vi "rsscope_core_global.vi"() -> ()   [LabVIEW 2014] (continued)
waveform types you can assign a suitable color table:\n              - each waveform of any channel\n              - a reference waveform\n              - the results of a mathematical function\n              - a stored measurement\n              - an xy-diagram\n              The following default color tables are provided:\n              - &apos;Temperature&apos;: shade of color changes gradually from blue (low temperature) to red (high temperature) with increasing cumulative occurance.\n              - &apos;False colors&apos;: color changes gradually in a wide color spectrum with increasing cumulative occurance.\n              - Spectrum: colors used to display the wave lengths of the light are assigned to the cumulative occurance. High cumulative occurance is displayed blue like high wave lenght.\n              - Single event: single events and very seldom events appear yellow, a higher cumulative occurance is shown with blue color. This view helps to indentify specific events.\n\nAvailable Repeated Capabilities:\nWfmSuffix: WfmNone, WfmC1W1, WfmC1W2, WfmC1W3, WfmC2W1, WfmC2W2, WfmC2W3, WfmC3W1, WfmC3W2, WfmC3W3, WfmC4W1, WfmC4W2, WfmC4W3, WfmMath1, WfmMath2, WfmMath3, WfmMath4, WfmRef1, WfmRef2, WfmRef3, WfmRef4, WfmXY1, WfmXY2, WfmXY3, WfmXY4, WfmMeas1, WfmMeas2, WfmMeas3, WfmMeas4, WfmMeas5, WfmMeas6, WfmMeas7, WfmMeas8, WfmSbus1, WfmSbus2, WfmSbus3, WfmSbus4, WfmD0, WfmD1, WfmD2, WfmD3, WfmD4, WfmD5, WfmD6, WfmD7, WfmD8, WfmD9, WfmD10, WfmD11, WfmD12, WfmD13, WfmD14, WfmD15, WfmMSO1, WfmMSO2, WfmMSO3, WfmMSO4, WfmTRK1, WfmTRK2, WfmTRK3, WfmTRK4, WfmTRK5, WfmTRK6, WfmTRK7, WfmTRK8, WfmSpectrum1, WfmSpectrum2, WfmSpectrum3, WfmSpectrum4, WfmSG1TL1, WfmSG1TL2, WfmSG2TL1, WfmSG2TL2, WfmSG3TL1, WfmSG3TL2, WfmSG4TL1, WfmSG4TL2, WfmEye1, WfmEye2, WfmEye3, WfmEye4, WfmZ1V1, WfmZ1V2, WfmZ1V3, WfmZ1V4, WfmZ1I1, WfmZ1I2, WfmZ1I3, WfmZ1I4, WfmZ2V1, WfmZ2V2, WfmZ2V3, WfmZ2V4, WfmZ2I1, WfmZ2I2, WfmZ2I3, WfmZ2I4, WfmDiff1, WfmDiff2, WfmCommon1, WfmCommon2, WfmTDRZ, WfmTDRH, WfmTDRR, WfmMath5, WfmMath6, WfmMath7, WfmMath8, WfmSpectrum5, WfmSpectrum6, WfmSpectrum7, WfmSpectrum8, WfmSG5TL1, WfmSG5TL2, WfmSG6TL1, WfmSG6TL2, WfmSG7TL1, WfmSG7TL2, WfmSG8TL1, WfmSG8TL2, WfmHP1, WfmHP2, WfmHP3, WfmHP4, WfmHP5, WfmHP6, WfmHP7, WfmHP8, WfmHP9, WfmHP10, WfmBathtub1, WfmBathMeas1, WfmStepResp1, WfmSRHist1, WfmSDHist1, WfmTJHist1, WfmDJHist1, WfmDDJHist1, WfmPJHist1, WfmRJOHist1, WfmSRTrack1, WfmTJTrack1, WfmDJTrack1, WfmDDJTrack1, WfmPJTrack1, WfmRJTrack1, WfmTJSpectrum1, WfmDDJSpectrum1, WfmPJSpectrum1, WfmRJSpectrum1, WfmSEye1, WfmBathtub2, WfmBathMeas2, WfmStepResp2, WfmSRHist2, WfmSDHist2, WfmTJHist2, WfmDJHist2, WfmDDJHist2, WfmPJHist2, WfmRJOHist2, WfmSRTrack2, WfmSDTrack2, WfmTJTrack2, WfmDDJTrack2, WfmPJTrack2, WfmRJTrack2, WfmTJSpectrum2, WfmDDJSpectrum2, WfmPJSpectrum2, WfmRJSpectrum2, WfmSEye2, WfmNBathtub1, WfmNBathMeas1, WfmTNHist1, WfmDNHist1, WfmDDNHist1, WfmPNHist1, WfmRNOTrack1, WfmTNTrack1, WfmDDNTrack1, WfmPNTrack1, WfmRNTrack1, WfmTNSpectrum1, WfmDDNSpectrum1, WfmPNSpectrum1, WfmRNSpectrum1, WfmNBathtub2, WfmNBathMeas2, WfmTNHist2, WfmDNHist2, WfmDDNHist2, WfmPNHist2, WfmRNOHist2, WfmTNTrack2, WfmDDNTrack2, WfmPNTrack2, WfmRNTrack2, WfmTNSpectrum2, WfmDDNSpectrum2, WfmPNSpectrum2, WfmRNSpectrum2, WfmPJDHist1, WfmBUJHist1, WfmRJHist1, WfmPJDTrack1, WfmPJDSpectrum1, WfmPJDHist2, WfmBUJHist2, WfmRJHist2, WfmPJDTrack2, WfmPJDSpectrum2, WfmPNDHist1, WfmBUNHist1, WfmRNHist1, WfmPNDTrack1, WfmPNDSpectrum1, WfmPNDHist2, WfmBUNHist2, WfmRNHist2, WfmPNDTrack2, WfmPNDSpectrum2\r\n\nRemote-control command(s):\nDISPlay:COLor:SIGNal<m>:ASSign"}, {"Level"=4, "Class Only"=FALSE, "Identifier"="RSSCOPE_ATTR_SIGNAL_COLOR", "Descriptive Name"="Signal Color", "Data Type"=5, "Command"="DISP:COL:SIGN{WfmSuffix}:COL", "Access"=2, "Range Table"="RsScope_rngSignalColor", "Read Callback"="", "Write Callback"="", "Supported Models"="", "Instrument Options"="", "Flags"=0, "Help"="Decimal value of the ARGB color. Use the color dialog box on the instrument to get the hex value of the color, and convert the hex value to a decimal value.\n0 is fully transparent black.\n4278190080 (dec) = FF000000 (hex) is opaque black.\n4294967295 (dec) = FFFFFFFF (hex) is opaque white.\n\nAvailable Repeated Capabilities:\nWfmSuffix: WfmNone, WfmC1W1, WfmC1W2, WfmC1W3, WfmC2W1, WfmC2W2, WfmC2W3, WfmC3W1, WfmC3W2, WfmC3W3, WfmC4W1, WfmC4W2, WfmC4W3, WfmMath1, WfmMath2, WfmMath3, WfmMath4, WfmRef1, WfmRef2, WfmRef3, WfmRef4, WfmXY1, WfmXY2, WfmXY3, WfmXY4, WfmMeas1, WfmMeas2, WfmMeas3, WfmMeas4, WfmMeas5, WfmMeas6, WfmMeas7, WfmMeas8, WfmSbus1, WfmSbus2, WfmSbus3, WfmSbus4, WfmD0, WfmD1, WfmD2, WfmD3, WfmD4, WfmD5, WfmD6, WfmD7, WfmD8, WfmD9, WfmD10, WfmD11, WfmD12, WfmD13, WfmD14, WfmD15, WfmMSO1, WfmMSO2, WfmMSO3, WfmMSO4, WfmTRK1, WfmTRK2, WfmTRK3, WfmTRK4, WfmTRK5, WfmTRK6, WfmTRK7, WfmTRK8, WfmSpectrum1, WfmSpectrum2, WfmSpectrum3, WfmSpectrum4, WfmSG1TL1, WfmSG1TL2, WfmSG2TL1, WfmSG2TL2, WfmSG3TL1, WfmSG3TL2, WfmSG4TL1, WfmSG4TL2, WfmEye1, WfmEye2, WfmEye3, WfmEye4, WfmZ1V1, WfmZ1V2, WfmZ1V3, WfmZ1V4, WfmZ1I1, WfmZ1I2, WfmZ1I3, WfmZ1I4, WfmZ2V1, WfmZ2V2, WfmZ2V3, WfmZ2V4, WfmZ2I1, WfmZ2I2, WfmZ2I3, WfmZ2I4, WfmDiff1, WfmDiff2, WfmCommon1, WfmCommon2, WfmTDRZ, WfmTDRH, WfmTDRR, WfmMath5, WfmMath6, WfmMath7, WfmMath8, WfmSpectrum5, WfmSpectrum6, WfmSpectrum7, WfmSpectrum8, WfmSG5TL1, WfmSG5TL2, WfmSG6TL1, WfmSG6TL2, WfmSG7TL1, WfmSG7TL2, WfmSG8TL1, WfmSG8TL2, WfmHP1, WfmHP2, WfmHP3, WfmHP4, WfmHP5, WfmHP6, WfmHP7, WfmHP8, WfmHP9, WfmHP10, WfmBathtub1, WfmBathMeas1, WfmStepResp1, WfmSRHist1, WfmSDHist1, WfmTJHist1, WfmDJHist1, WfmDDJHist1, WfmPJHist1, WfmRJOHist1, WfmSRTrack1, WfmTJTrack1, WfmDJTrack1, WfmDDJTrack1, WfmPJTrack1, WfmRJTrack1, WfmTJSpectrum1, WfmDDJSpectrum1, WfmPJSpectrum1, WfmRJSpectrum1, WfmSEye1, WfmBathtub2, WfmBathMeas2, WfmStepResp2, WfmSRHist2, WfmSDHist2, WfmTJHist2, WfmDJHist2, WfmDDJHist2, WfmPJHist2, WfmRJOHist2, WfmSRTrack2, WfmSDTrack2, WfmTJTrack2, WfmDDJTrack2, WfmPJTrack2, WfmRJTrack2, WfmTJSpectrum2, WfmDDJSpectrum2, WfmPJSpectrum2, WfmRJSpectrum2, WfmSEye2, WfmNBathtub1, WfmNBathMeas1, WfmTNHist1, WfmDNHist1, WfmDDNHist1, WfmPNHist1, WfmRNOTrack1, WfmTNTrack1, WfmDDNTrack1, WfmPNTrack1, WfmRNTrack1, WfmTNSpectrum1, WfmDDNSpectrum1, WfmPNSpectrum1, WfmRNSpectrum1, WfmNBathtub2, WfmNBathMeas2, WfmTNHist2, WfmDNHist2, WfmDDNHist2, WfmPNHist2, WfmRNOHist2, WfmTNTrack2, WfmDDNTrack2, WfmPNTrack2, WfmRNTrack2, WfmTNSpectrum2, WfmDDNSpectrum2, WfmPNSpectrum2, WfmRNSpectrum2, WfmPJDHist1, WfmBUJHist1, WfmRJHist1, WfmPJDTrack1, WfmPJDSpectrum1, WfmPJDHist2, WfmBUJHist2, WfmRJHist2, WfmPJDTrack2, WfmPJDSpectrum2, WfmPNDHist1, WfmBUNHist1, WfmRNHist1, WfmPNDTrack1, WfmPNDSpectrum1, WfmPNDHist2, WfmBUNHist2, WfmRNHist2, WfmPNDTrack2, WfmPNDSpectrum2\r\n\nRemote-control command(s):\nDISPlay:COLor:SIGNal<m>:COLor"}, {"Level"=2, "Class Only"=TRUE, "Identifier"="", "Descriptive Name"="Color Tables", "Data Type"=0, "Command"="", "Access"=0, "Range Table"="", "Read Callback"="", "Write Callback"="", "Supported Models"="", "Instrument Options"="", "Flags"=0, "Help"="Configuration for color tables."}, {"Level"=3, "Class Only"=FALSE, "Identifier"="RSSCOPE_ATTR_ADD_COLOR_TABLE", "Descriptive Name"="Add Color Table", "Data Type"=2, "Command"="DISP:COL:PAL:ADD", "Access"=1, "Range Table"="", "Read Callback"="", "Write Callback"="", "Supported Models"="", "Instrument Options"="", "Flags"=0, "Help"="Adds a new color table with the specified name.\n\nAvailable Repeated Capabilities:\nNone\n\nRemote-control command(s):\nDISPlay:COLor:PALette:ADD"}, {"Level"=3, "Class Only"=FALSE, "Identifier"="RSSCOPE_ATTR_REMOVE_COLOR_TABLE", "Descriptive Name"="Remove Color Table", "Data Type"=2, "Command"="DISP:COL:PAL:REM", "Access"=1, "Range Table"="", "Read Callback"="", "Write Callback"="", "Supported Models"="", "Instrument Options"="", "Flags"=0, "Help"="Removes the specified color table.\n\nAvailable Repeated Capabilities:\nNone\n\nRemote-control command(s):\nDISPlay:COLor:PALette:REMove"}, {"Level"=3, "Class Only"=FALSE, "Identifier"="RSSCOPE_ATTR_COLOR_TABLE_COUNT", "Descriptive Name"="Color Table Count", "Data Type"=0, "Command"="DISP:COL:PAL:COUN?", "Access"=0, "Range Table"="", "Read Callback"="", "Write Callback"="", "Supported Models"="", "Instrument Options"="", "Flags"=0, "Help"="Queries the number of configured color maps.\n\nAvailable Repeated Capabilities:\nNone\n\nRemote-control command(s):\nDISPlay:COLor:PALette:COUNt?"}, {"Level"=3, "Class Only"=FALSE, "Identifier"="RSSCOPE_ATTR_COLOR_TABLE_APPEND_NEW_ROW", "Descriptive Name"="Color Table Append New Row", "Data Type"=2, "Command"="DISP:COL:PAL:POIN:ADD", "Access"=1, "Range Table"="", "Read Callback"="", "Write Callback"="", "Supported Models"="", "Instrument Options"="", "Flags"=0, "Help"="Appends a new row at the end of the color table.\n\nAvailable Repeated Capabilities:\nNone\n\nRemote-control command(s):\nDISPlay:COLor:PALette:POINt:ADD"}, {"Level"=2, "Class Only"=TRUE, "Identifier"="", "Descriptive Name"="Diagram Layout", "Data Type"=0, "Command"="", "Access"=0, "Range Table"="", "Read Callback"="", "Write Callback"="", "Supported Models"="", "Instrument Options"="", "Flags"=0, "Help"="Configuration for diagram layout."}, {"Level"=3, "Class Only"=FALSE, "Identifier"="RSSCOPE_ATTR_DIAGRAM_SHOW_GRID", "Descriptive Name"="Diagram Show Grid", "Data Type"=3, "Command"="DISP:DIAG:GRID", "Access"=2, "Range Table"="", "Read Callback"="", "Write Callback"="", "Supported Models"="", "Instrument Options"="", "Flags"=0, "Help"="If enabled, a grid is displayed in the diagram area.\n\nAvailable Repeated Capabilities:\nNone\n\nRemote-control command(s):\nDISPlay:DIAGram:GRID"}, {"Level"=3, "Class Only"=FALSE, "Identifier"="RSSCOPE_ATTR_DIAGRAM_SHOW_CROSSHAIR", "Descriptive Name"="Diagram Show Crosshair", "Data Type"=3, "Command"="DISP:DIAG:CROS", "Access"=2, "Range Table"="", "Read Callback"="", "Write Callback"="", "Supported Models"="", "Instrument Options"="", "Flags"=0, "Help"="If selected, a crosshair is displayed in the diagram area. A crosshair allows you to select a specific data point by its co-ordinates.\n\nAvailable Repeated Capabilities:\nNone\n\nRemote-control command(s):\nDISPlay:DIAGram:CROSshair"}, {"Level"=3, "Class Only"=FALSE, "Identifier"="RSSCOPE_ATTR_DIAGRAM_SHOW_LABELS", "Descriptive Name"="Diagram Show Labels", "Data Type"=3, "Command"="DISP:DIAG:LAB", "Access"=2, "Range Table"="", "Read Callback"="", "Write Callback"="", "Supported Models"="", "Instrument Options"="", "Flags"=0, "Help"="If enabled, labels mark values on the x- and y-axes in specified intervals in the diagram.\n\nAvailable Repeated Capabilities:\nNone\n\nRemote-control command(s):\nDISPlay:DIAGram:LABels"}, {"Level"=3, "Class Only"=FALSE, "Identifier"="RSSCOPE_ATTR_DIAGRAM_SHOW_TAB_TITLES", "Descriptive Name"="Diagram Show Tab Titles", "Data Type"=3, "Command"="DISP:DIAG:TITL", "Access"=2, "Range Table"="", "Read Callback"="", "Write Callback"="", "Supported Models"="", "Instrument Options"="", "Flags"=0, "Help"="If enabled, the tab titles of all diagrams are displayed: &apos;Diagram1&apos;, &apos;Diagram2&apos;, ...\nIf disabled, the tab titles are not shown except for those in a tabbed diagram. In tabbed diagrams, the tab titles are required to change the tabs.\n\nAvailable Repeated Capabilities:\nNone\n\nRemote-control command(s):\nDISPlay:DIAGram:TITLe"}, {"Level"=3, "Class Only"=FALSE, "Identifier"="RSSCOPE_ATTR_DIAGRAM_KEEP_Y_GRID_FIXED", "Descriptive Name"="Diagram Keep Y-grid Fixed", "Data Type"=3, "Command"="DISP:DIAG:YFIX", "Access"=2, "Range Table"="", "Read Callback"="", "Write Callback"="", "Supported Models"="", "Instrument Options"="", "Flags"=0, "Help"="If enabled, the horizontal grid lines remain in their position when the position of the curve is changed. Only the values at the grid lines are adapted. This reflects the behavior of traditional oscilloscopes.\n\nAvailable Repeated Capabilities:\nNone\n\nRemote-control command(s):\nDISPlay:DIAGram:YFIXed"}, {"Level"=3, "Class Only"=FALSE, "Identifier"="RSSCOPE_ATTR_DIAGRAM_KEEP_X_GRID_FIXED", "Descriptive Name"="Diagram Keep X-grid Fixed", "Data Type"=3, "Command"="DISP:DIAG:XFIX", "Access"=2, "Range Table"="", "Read Callback"="", "Write Callback"="", "Supported Models"="", "Instrument Options"="", "Flags"=0, "Help"="If enabled, the vertical grid lines remain in their position when the horizontal position is changed. Only the values at the grid lines are adapted.\n\nAvailable Repeated Capabilities:\nNone\n\nRemote-control command(s):\nDISPlay:DIAGram:XFIXed"}, {"Level"=3, "Class Only"=FALSE, "Identifier"="RSSCOPE_ATTR_DIAGRAM_SHOW_FINE_GRID_SCALE", "Descriptive Name"="Diagram Show Fine Grid Scale", "Data Type"=3, "Command"="DISP:DIAG:FIN", "Access"=2, "Range Table"="", "Read Callback"="", "Write Callback"="", "Supported Models"="", "Instrument Options"="", "Flags"=0, "Help"="Configures fine grid scaling.\n\nAvailable Repeated Capabilities:\nNone\n\nRemote-control command(s):\nDISPlay:DIAGram:FINegrid"}, {"Level"=3, "Class Only"=FALSE, "Identifier"="RSSCOPE_ATTR_SIGNAL_BAR_STATE", "Descriptive Name"="Signal Bar State", "Data Type"=3, "Command"="DISP:SIGB:STAT", "Access"=2, "Range Table"="", "Read Callback"="", "Write Callback"="", "Supported Models"="", "Instrument Options"="", "Flags"=0, "Help"="If enabled, the signal bar is displayed in the diagram area.\n\nAvailable Repeated Capabilities:\nNone\n\nRemote-control command(s):\nDISPlay:SIGBar[:STATe]"}, {"Level"=3, "Class Only"=FALSE, "Identifier"="RSSCOPE_ATTR_SIGNAL_BAR_POSITION", "Descriptive Name"="Signal Bar Position", "Data Type"=0, "Command"="DISP:SIGB:POS", "Access"=2, "Range Table"="rsscope_rngSignalBarPostion", "Read Callback"="", "Write Callback"="", "Supported Models"="", "Instrument Options"="", "Flags"=0, "Help"="The signal bar can be placed vertically at the right (default position) or at the left, or horizontally at the top, bottom or center of the diagram to ensure best visibility of the waveforms.\n\nAvailable Repeated Capabilities:\nNone\n\nRemote-control command(s):\nDISPlay:SIGBar:POSition"}, {"Level"=3, "Class Only"=FALSE, "Identifier"="RSSCOPE_ATTR_SIGNAL_BAR_AUTO_HIDE", "Descriptive Name"="Signal Bar Auto Hide", "Data Type"=3, "Command"="DISP:SIGB:HIDE:AUTO", "Access"=2, "Range Table"="", "Read Callback"="", "Write Callback"="", "Supported Models"="", "Instrument Options"="", "Flags"=0, "Help"="If enabled, the signal bar disappears automatically after some time, similar to the Windows task bar. With the commands DISPlay:SIGBar:HIDE:TIME and DISPlay:SIGBar:HIDE:OPACity, you can define when and how the signal bar hides.\nThe signal bar reappears if you tap it, or if an action changes the content of the bar.\n\nAvailable Repeated Capabilities:\nNone\n\nRemote-control command(s):\nDISPlay:SIGBar:HIDE[:AUTO]"}, {"Level"=3, "Class Only"=FALSE, "Identifier"="RSSCOPE_ATTR_SIGNAL_BAR_HIDE_TIME", "Descriptive Name"="Signal Bar Hide Time", "Data Type"=1, "Command"="DISP:SIGB:HIDE:TIME", "Access"=2, "Range Table"="rsscope_rngSignalBarHideTime", "Read Callback"="", "Write Callback"="", "Supported Models"="", "Instrument Options"="", "Flags"=0, "Help"="Sets the time when the signal bar is faded out if DISPlay:SIGBar:HIDE[:AUTO] is &apos;ON&apos;\n\nAvailable Repeated Capabilities:\nNone\n\nRemote-control command(s):\nDISPlay:SIGBar:HIDE:TIME"}, {"Level"=3, "Class Only"=FALSE, "Identifier"="RSSCOPE_ATTR_SIGNAL_BAR_HIDE_HEAD", "Descriptive Name"="Signal Bar Hide Head", "Data Type"=3, "Command"="DISP:SIGB:HIDE:HEAD", "Access"=2, "Range Table"="", "Read Callback"="", "Write Callback"="", "Supported Models"="", "Instrument Options"="", "Flags"=0, "Help"="If enabled, the &apos;Auto hide&apos; function hides also the horizontal and trigger label at the top of the signal bar.\n\nAvailable Repeated Capabilities:\nNone\n\nRemote-control command(s):\nDISPlay:SIGBar:HIDE:HEAD"}, {"Level"=3, "Class Only"=FALSE, "Identifier"="RSSCOPE_ATTR_SIGNAL_BAR_HIDING_TRANSPARENCY", "Descriptive Name"="Signal Bar Hiding Transparency", "Data Type"=1, "Command"="DISP:SIGB:HIDE:TRAN", "Access"=2, "Range Table"="rsscope_rngSignalBarHidingTransparency", "Read Callback"="", "Write Callback"="", "Supported Models"="", "Instrument Options"="", "Flags"=0, "Help"="Sets the opacity, or transparency, of the signal bar. The minimum value is 30% for the least visibility of the signal bar, the maximum value is 80%.\n\nAvailable Repeated Capabilities:\nNone\n\nRemote-control command(s):\nDISPlay:SIGBar:HIDE:TRANsparency"}, {"Level"=3, "Class Only"=FALSE, "Identifier"="RSSCOPE_ATTR_SIGNAL_BAR_BORDER_COLOR", "Descriptive Name"="Signal Bar Border Color", "Data Type"=0, "Command"="DISP:SIGB:COL:BORD", "Access"=2, "Range Table"="", "Read Callback"="", "Write Callback"="", "Supported Models"="", "Instrument Options"="", "Flags"=0, "Help"="Defines the color of the signal bar border.\n\nAvailable Repeated Capabilities:\nNone\n\nRemote-control command(s):\nDISPlay:SIGBar:COLor:BORDer"}, {"Level"=3, "Class Only"=FALSE, "Identifier"="RSSCOPE_ATTR_SIGNAL_BAR_FILL_COLOR", "Descriptive Name"="Signal Bar Fill Color", "Data Type"=0, "Command"="DISP:SIGB:COL:FILL", "Access"=2, "Range Table"="", "Read Callback"="", "Write Callback"="", "Supported Models"="", "Instrument Options"="", "Flags"=0, "Help"="Define the fill color of the signal bar.\n\nAvailable Repeated Capabilities:\nNone\n\nRemote-control command(s):\nDISPlay:SIGBar:COLor:FILL"}, {"Level"=3, "Class Only"=FALSE, "Identifier"="RSSCOPE_ATTR_RESULT_BOX_POSITION", "Descriptive Name"="Result Box Position", "Data Type"=0, "Command"="DISP:RES:DEF", "Access"=2, "Range Table"="rsscope_rngResultBoxPosition", "Read Callback"="", "Write Callback"="", "Supported Models"="", "Instrument Options"="", "Flags"=0, "Help"="Defines where a new result box opens.\n\nAvailable Repeated Capabilities:\nNone\n\nRemote-control command(s):\nDISPlay:RESultboxes:DEFaultpos"}, {"Level"=3, "Class Only"=FALSE, "Identifier"="RSSCOPE_ATTR_REMOVE_DIAGRAM", "Descriptive Name"="Remove Diagram", "Data Type"=2, "Command"="LAY:REM", "Access"=1, "Range Table"="", "Read Callback"="", "Write Callback"="", "Supported Models"="", "Instrument Options"="", "Flags"=0, "Help"="Removes diagram\n\nAvailable Repeated Capabilities:\nNone\n\nRemote-control command(s):\nLAYout:REMove"}, {"Level"=3, "Class Only"=FALSE, "Identifier"="RSSCOPE_ATTR_DISPLAY_DIAGRAM", "Descriptive Name"="Display Diagram", "Data Type"=2, "Command"="LAY:SHOW", "Access"=1, "Range Table"="", "Read Callback"="", "Write Callback"="", "Supported Models"="", "Instrument Options"="", "Flags"=0, "Help"="Displays diagram.\n\nAvailable Repeated Capabilities:\nNone\n\nRemote-control command(s):\nLAYout:SHOW"}, {"Level"=3, "Class Only"=FALSE, "Identifier"="RSSCOPE_ATTR_REMOVE_WAVEFORM_FROM_DIAGRAM", "Descriptive Name"="Remove Waveform From Diagram", "Data Type"=0, "Command"="LAY:SIGN:UNAS", "Access"=1, "Range Table"="rsscope_rngWaveformParameter", "Read Callback"="", "Write Callback"="", "Supported Models"="", "Instrument Options"="", "Flags"=0, "Help"="Removes the specified waveform from the diagram.\n\nAvailable Repeated Capabilities:\nNone\n\nRemote-control command(s):\nLAYout:SIGNal:UNASsign"}, {"Level"=2, "Class Only"=TRUE, "Identifier"="", "Descriptive Name"="Waveform Label", "Data Type"=0, "Command"="", "Access"=0, "Range Table"="", "Read Callback"="", "Write Callback"="", "Supported Models"="", "Instrument Options"="", "Flags"=0, "Help"="Attributes which configures labels of waveforms."}, {"Level"=3, "Class Only"=FALSE, "Identifier"="RSSCOPE_ATTR_SELECTED_LABEL_NAME", "Descriptive Name"="Selected Label Name", "Data Type"=2, "Command"="", "Access"=2, "Range Table"="", "Read Callback"="", "Write Callback"="", "Supported Models"="", "Instrument Options"="", "Flags"=0, "Help"="This attribute selects the label name used for following attributes.\n\nAvailable Repeated Capabilities:\nNone\n\nRemote-control command(s):\ncmd"}, {"Level"=3, "Class Only"=FALSE, "Identifier"="RSSCOPE_ATTR_SELECTED_LABEL_SOURCE", "Descriptive Name"="Selected Label Source", "Data Type"=0, "Command"="", "Access"=2, "Range Table"="rsscope_rngWaveformParameter", "Read Callback"="", "Write Callback"="", "Supported Models"="", "Instrument Options"="", "Flags"=0, "Help"="Sets selector repeated capability Source.\n\nAvailable Repeated Capabilities:\nNone\n\nRemote-control command(s):\n"}, {"Level"=3, "Class Only"=FALSE, "Identifier"="RSSCOPE_ATTR_LABEL_SHOW", "Descriptive Name"="Label Show", "Data Type"=3, "Command"="DISP:SIGN:LAB:SHOW", "Access"=2, "Range Table"="", "Read Callback"="rsscope_FormatLabelSourceBoolean_ReadCallback.vi", "Write Callback"="rsscope_FormatLabelSourceBoolean_WriteCallback.vi", "Supported Models"="", "Instrument Options"="", "Flags"=0, "Help"="Selects the source for the label display and enables it.\n\nAvailable Repeated Capabilities:\nNone\n\nRemote-control command(s):\nDISPlay:SIGNal:LABel:SHOW"}, {"Level"=3, "Class Only"=FALSE, "Identifier"="RSSCOPE_ATTR_WAVEFORM_LABEL_FONT_SIZE", "Descriptive Name"="Waveform Label Font Size", "Data Type"=0, "Command"="DISPlay:SIGNal:LABel:FONTsize", "Access"=2, "Range Table"="RsScope_rngWaveformLabelFontSize", "Read Callback"="", "Write Callback"="", "Supported Models"="", "Instrument Options"="", "Flags"=0, "Help"="Sets the font size of waveform labels.\n\nAvailable Repeated Capabilities:\nNone\n\nRemote-control command(s):\nDISPlay:SIGNal:LABel:FONTsize"}, {"Level"=2, "Class Only"=TRUE, "Identifier"="", "Descriptive Name"="Zoom", "Data Type"=0, "Command"="", "Access"=0, "Range Table"="", "Read Callback"="", "Write Callback"="", "Supported Models"="", "Instrument Options"="", "Flags"=0, "Help"="The zoom attributes allow you to magnify a specific section of the diagram in order to view more details. You can define several zoom areas for the same diagram and even couple them, or you use the hardware zoom."}, {"Level"=3, "Class Only"=FALSE, "Identifier"="RSSCOPE_ATTR_DIAGRAM_ZOOM_OVERLAY", "Descriptive Name"="Diagram Zoom Overlay", "Data Type"=3, "Command"="LAY:ZOOM:ONED", "Access"=2, "Range Table"="", "Read Callback"="", "Write Callback"="", "Supported Models"="", "Instrument Options"="", "Flags"=0, "Help"="Shows all zooms of a diagram in one zoom window.\n\nAvailable Repeated Capabilities:\nNone\n\nRemote-control command(s):\nLAYout:ZOOM:ONEDiagram"}, {"Level"=2, "Class Only"=TRUE, "Identifier"="", "Descriptive Name"="XY Diagram", "Data Type"=0, "Command"="", "Access"=0, "Range Table"="", "Read Callback"="", "Write Callback"="", "Supported Models"="", "Instrument Options"="", "Flags"=0, "Help"="Configuration for XY diagrams."}, {"Level"=3, "Class Only"=FALSE, "Identifier"="RSSCOPE_ATTR_XY_DIAGRAM_STATE", "Descriptive Name"="XY Diagram State", "Data Type"=3, "Command"="WAV{XYDiagram}:XYC:STAT", "Access"=2, "Range Table"="", "Read Callback"="", "Write Callback"="", "Supported Models"="", "Instrument Options"="", "Flags"=0, "Help"="Activates an XY-waveform.\n\nAvailable Repeated Capabilities:\nXYDiagram: XY1, XY2, XY3, XY4\r\n\nRemote-control command(s):\nWAVeform<m>:XYCurve:STATe"}, {"Level"=3, "Class Only"=FALSE, "Identifier"="RSSCOPE_ATTR_XY_DIAGRAM_RATIO", "Descriptive Name"="XY Diagram Ratio", "Data Type"=3, "Command"="WAV{XYDiagram}:XYC:RAT", "Access"=2, "Range Table"="", "Read Callback"="", "Write Callback"="", "Supported Models"="", "Instrument Options"="", "Flags"=0, "Help"="If enabled, the x- and y-axes maintain a constant ratio in the diagram.\n\nAvailable Repeated Capabilities:\nXYDiagram: XY1, XY2, XY3, XY4\r\n\nRemote-control command(s):\nWAVeform<m>:XYCurve:RATio"}, {"Level"=3, "Class Only"=FALSE, "Identifier"="RSSCOPE_ATTR_SWAP_XY_DIAGRAM", "Descriptive Name"="Swap XY Diagram", "Data Type"=4, "Command"="WAV{XYDiagram}:XYC:SWAP", "Access"=1, "Range Table"="", "Read Callback"="", "Write Callback"="", "Supported Models"="", "Instrument Options"="", "Flags"=0, "Help"="Replaces the source of the x-axis with the source of the y-axis and vice versa.\n\nAvailable Repeated Capabilities:\nXYDiagram: XY1, XY2, XY3, XY4\r\n\nRemote-control command(s):\nWAVeform<m>:XYCurve:SWAP"}, {"Level"=3, "Class Only"=FALSE, "Identifier"="RSSCOPE_ATTR_XY_DIAGRAM_X_SOURCE", "Descriptive Name"="XY Diagram X Source", "Data Type"=0, "Command"="WAV{XYDiagram}:XYC:XSO", "Access"=2, "Range Table"="rsscope_rngWaveformParameterXY", "Read Callback"="", "Write Callback"="", "Supported Models"="", "Instrument Options"="", "Flags"=0, "Help"="Defines the signal source that supplies the x-values of the XY-diagram.\n\nAvailable Repeated Capabilities:\nXYDiagram: XY1, XY2, XY3, XY4\r\n\nRemote-control command(s):\nWAVeform<m>:XYCurve:XSOurce"}, {"Level"=3, "Class Only"=FALSE, "Identifier"="RSSCOPE_ATTR_XY_DIAGRAM_Y_SOURCE", "Descriptive Name"="XY Diagram Y Source", "Data Type"=0, "Command"="WAV{XYDiagram}:XYC:YSO", "Access"=2, "Range Table"="rsscope_rngWaveformParameterXY", "Read Callback"="", "Write Callback"="", "Supported Models"="", "Instrument Options"="", "Flags"=0, "Help"="Defines the signal source that supplies the y-values of the XY-diagram.\n\nAvailable Repeated Capabilities:\nXYDiagram: XY1, XY2, XY3, XY4\r\n\nRemote-control command(s):\nWAVeform<m>:XYCurve:YSOurce"}, {"Level"=2, "Class Only"=TRUE, "Identifier"="", "Descriptive Name"="History", "Data Type"=0, "Command"="", "Access"=0, "Range Table"="", "Read Callback"="", "Write Callback"="", "Supported Models"="", "Instrument Options"="", "Flags"=0, "Help"="This class contains functions for history viewing and information."}, {"Level"=3, "Class Only"=FALSE, "Identifier"="RSSCOPE_ATTR_HISTORY_GET_ACQUISITIONS_COUNT", "Descriptive Name"="History Get Acquisitions Count", "Data Type"=0, "Command"="ACQ:AVA?", "Access"=0, "Range Table"="", "Read Callback"="", "Write Callback"="", "Supported Models"="", "Instrument Options"="", "Flags"=0, "Help"="Returns the number of acquisitions currently saved in the memory.\n\nAvailable Repeated Capabilities:\nNone\n\nRemote-control command(s):\nACQuire:AVAilable?"}, {"Level"=3, "Class Only"=TRUE, "Identifier"="", "Descriptive Name"="Channel", "Data Type"=0, "Command"="", "Access"=0, "Range Table"="", "Read Callback"="", "Write Callback"="", "Supported Models"="", "Instrument Options"="", "Flags"=0, "Help"="Configures Display History properties."}, {"Level"=4, "Class Only"=TRUE, "Identifier"="", "Descriptive Name"="Waveform", "Data Type"=0, "Command"="", "Access"=0, "Range Table"="", "Read Callback"="", "Write Callback"="", "Supported Models"="", "Instrument Options"="", "Flags"=0, "Help"="Configures History Waveform properties."}, {"Level"=5, "Class Only"=FALSE, "Identifier"="RSSCOPE_ATTR_HISTORY_STATE", "Descriptive Name"="History State", "Data Type"=3, "Command"="CHAN{Channel}:WAV{Waveform}:HIST", "Access"=2, "Range Table"="", "Read Callback"="", "Write Callback"="", "Supported Models"="", "Instrument Options"="", "Flags"=0, "Help"="Enables or disables the history display.\n\nAvailable Repeated Capabilities:\nChannel: CH1, CH2, CH3, CH4, CHExt\r\nWaveform: W0, W1, W2, W3\r\n\nRemote-control command(s):\nCHANnel<m>[:WAVeform<n>]:HISTory[:STATe]"}, {"Level"=5, "Class Only"=FALSE, "Identifier"="RSSCOPE_ATTR_HISTORY_START_INDEX", "Descriptive Name"="History Start Index", "Data Type"=0, "Command"="CHAN{Channel}:WAV{Waveform}:HIST:STAR", "Access"=2, "Range Table"="", "Read Callback"="", "Write Callback"="", "Supported Models"="", "Instrument Options"="", "Flags"=0, "Help"="Sets the start point for the history replay.\nNote: The &apos;Start index&apos; is always negative.\n\nAvailable Repeated Capabilities:\nChannel: CH1, CH2, CH3, CH4, CHExt\r\nWaveform: W0, W1, W2, W3\r\n\nRemote-control command(s):\nCHANnel<m>[:WAVeform<n>]:HISTory:STARt"}, {"Level"=5, "Class Only"=FALSE, "Identifier"="RSSCOPE_ATTR_HISTORY_STOP_INDEX", "Descriptive Name"="History Stop Index", "Data Type"=0, "Command"="CHAN{Channel}:WAV{Waveform}:HIST:STOP", "Access"=2, "Range Table"="", "Read Callback"="", "Write Callback"="", "Supported Models"="", "Instrument Options"="", "Flags"=0, "Help"="Sets the end point for the history viewer.\nNote: The newest acquisition always has the index &apos;0&apos;.\n\nAvailable Repeated Capabilities:\nChannel: CH1, CH2, CH3, CH4, CHExt\r\nWaveform: W0, W1, W2, W3\r\n\nRemote-control command(s):\nCHANnel<m>[:WAVeform<n>]:HISTory:STOP"}, {"Level"=5, "Class Only"=FALSE, "Identifier"="RSSCOPE_ATTR_HISTORY_ACQUISITION_VIEW", "Descriptive Name"="History Acquisition View", "Data Type"=0, "Command"="CHAN{Channel}:WAV{Waveform}:HIST:CURR", "Access"=2, "Range Table"="", "Read Callback"="", "Write Callback"="", "Supported Models"="", "Instrument Options"="", "Flags"=0, "Help"="Selects a particular acquisition in the memory to display it.\n\nAvailable Repeated Capabilities:\nChannel: CH1, CH2, CH3, CH4, CHExt\r\nWaveform: W0, W1, W2, W3\r\n\nRemote-control command(s):\nCHANnel<m>[:WAVeform<n>]:HISTory:CURRent"}, {"Level"=5, "Class Only"=FALSE, "Identifier"="RSSCOPE_ATTR_HISTORY_ACQUISITION_TIME", "Descriptive Name"="History Acquisition Time", "Data Type"=1, "Command"="CHAN{Channel}:WAV{Waveform}:HIST:TPAC", "Access"=2, "Range Table"="rsscope_rngHistAcqTime", "Read Callback"="", "Write Callback"="", "Supported Models"="", "Instrument Options"="", "Flags"=0, "Help"="Sets the display time for one acquisition.\n\nAvailable Repeated Capabilities:\nChannel: CH1, CH2, CH3, CH4, CHExt\r\nWaveform: W0, W1, W2, W3\r\n\nRemote-control command(s):\nCHANnel<m>[:WAVeform<n>]:HISTory:TPACq"}, {"Level"=5, "Class Only"=FALSE, "Identifier"="RSSCOPE_ATTR_HISTORY_AUTO_REPEAT", "Descriptive Name"="History Auto Repeat", "Data Type"=3, "Command"="CHAN{Channel}:WAV{Waveform}:HIST:REPL", "Access"=2, "Range Table"="", "Read Callback"="", "Write Callback"="", "Supported Models"="", "Instrument Options"="", "Flags"=0, "Help"="Sets if the replay of the history waveform sequence repeats automatically.\n\nAvailable Repeated Capabilities:\nChannel: CH1, CH2, CH3, CH4, CHExt\r\nWaveform: W0, W1, W2, W3\r\n\nRemote-control command(s):\nCHANnel<m>[:WAVeform<n>]:HISTory:REPLay"}, {"Level"=5, "Class Only"=FALSE, "Identifier"="RSSCOPE_ATTR_HISTORY_PLAYBACK", "Descriptive Name"="History Playback", "Data Type"=4, "Command"="CHAN{Channel}:WAV{Waveform}:HIST:PLAY", "Access"=1, "Range Table"="", "Read Callback"="", "Write Callback"="", "Supported Models"="", "Instrument Options"="", "Flags"=0, "Help"="Starts and stops the replay of the history waveforms.\n\nAvailable Repeated Capabilities:\nChannel: CH1, CH2, CH3, CH4, CHExt\r\nWaveform: W0, W1, W2, W3\r\n\nRemote-control command(s):\nCHANnel<m>[:WAVeform<n>]:HISTory:PLAY"}, {"Level"=5, "Class Only"=FALSE, "Identifier"="RSSCOPE_ATTR_HISTORY_ABSOLUTE_TIME_STAMP", "Descriptive Name"="History Absolute Time Stamp", "Data Type"=2, "Command"="CHAN{Channel}:WAV{Waveform}:HIST:TSAB?", "Access"=0, "Range Table"="", "Read Callback"="", "Write Callback"="", "Supported Models"="", "Instrument Options"="", "Flags"=0, "Help"="Returns the abolsute daytime of the current acquisition that is shown in the history viewer\n\nAvailable Repeated Capabilities:\nChannel: CH1, CH2, CH3, CH4, CHExt\r\nWaveform: W0, W1, W2, W3\r\n\nRemote-control command(s):\nCHANnel<m>[:WAVeform<n>]:HISTory:TSABsolute?"}, {"Level"=5, "Class Only"=FALSE, "Identifier"="RSSCOPE_ATTR_HISTORY_RELATIVE_TIME_STAMP", "Descriptive Name"="History Relative Time Stamp", "Data Type"=2, "Command"="CHAN{Channel}:WAV{Waveform}:HIST:TSR?", "Access"=0, "Range Table"="", "Read Callback"="", "Write Callback"="", "Supported Models"="", "Instrument Options"="", "Flags"=0, "Help"="Returns the relative time of the current acquisition - the time difference to the newest acquisition (index = 0).\n\nAvailable Repeated Capabilities:\nChannel: CH1, CH2, CH3, CH4, CHExt\r\nWaveform: W0, W1, W2, W3\r\n\nRemote-control command(s):\nCHANnel<m>[:WAVeform<n>]:HISTory:TSRelative?"}, {"Level"=5, "Class Only"=FALSE, "Identifier"="RSSCOPE_ATTR_HISTORY_TIME_REFERENCE", "Descriptive Name"="History Time Reference", "Data Type"=1, "Command"="CHAN{Channel}:WAV{Waveform}:HIST:TSRR?", "Access"=0, "Range Table"="", "Read Callback"="", "Write Callback"="", "Supported Models"="", "Instrument Options"="", "Flags"=0, "Help"="Returns the relative time of the currently selected acquisition and the internal reference time (horizontal alignment) in history view with respect to the acquisition with index 0.\n\nAvailable Repeated Capabilities:\nChannel: CH1, CH2, CH3, CH4, CHExt\r\nWaveform: W0, W1, W2, W3\r\n\nRemote-control command(s):\nCHANnel<m>[:WAVeform<n>]:HISTory:TSRReference?"}, {"Level"=5, "Class Only"=FALSE, "Identifier"="RSSCOPE_ATTR_HISTORY_DATE", "Descriptive Name"="History Date", "Data Type"=2, "Command"="CHAN{Channel}:WAV{Waveform}:HIST:TSD?", "Access"=0, "Range Table"="", "Read Callback"="", "Write Callback"="", "Supported Models"="", "Instrument Options"="", "Flags"=0, "Help"="Returns the date of the current acquisition that is shown in the history viewer.\n\nAvailable Repeated Capabilities:\nChannel: CH1, CH2, CH3, CH4, CHExt\r\nWaveform: W0, W1, W2, W3\r\n\nRemote-control command(s):\nCHANnel<m>[:WAVeform<n>]:HISTory:TSDate?"}, {"Level"=1, "Class Only"=TRUE, "Identifier"="", "Descriptive Name"="Data Management", "Data Type"=0, "Command"="", "Access"=0, "Range Table"="", "Read Callback"="", "Write Callback"="", "Supported Models"="", "Instrument Options"="", "Flags"=0, "Help"="Mass memory, save and load"}, {"Level"=2, "Class Only"=FALSE, "Identifier"="RSSCOPE_ATTR_SAVE", "Descriptive Name"="Save", "Data Type"=0, "Command"="*SAV", "Access"=1, "Range Table"="", "Read Callback"="", "Write Callback"="", "Supported Models"="", "Instrument Options"="", "Flags"=0, "Help"="Saves settings.\n\nAvailable Repeated Capabilities:\nNone\n\nRemote-control command(s):\n*SAV"}, {"Level"=2, "Class Only"=FALSE, "Identifier"="RSSCOPE_ATTR_RECALL", "Descriptive Name"="Recall", "Data Type"=0, "Command"="*RCL", "Access"=1, "Range Table"="", "Read Callback"="", "Write Callback"="", "Supported Models"="", "Instrument Options"="", "Flags"=0, "Help"="Recalls settings.\n\nAvailable Repeated Capabilities:\nNone\n\nRemote-control command(s):\n*RCL"}, {"Level"=2, "Class Only"=FALSE, "Identifier"="RSSCOPE_ATTR_DRIVES", "Descriptive Name"="Drives", "Data Type"=2, "Command"="MMEM:DRIV?", "Access"=0, "Range Table"="", "Read Callback"="", "Write Callback"="", "Supported Models"="", "Instrument Options"="", "Flags"=0, "Help"="Returns a list of the drives of the instrument.\n\nAvailable Repeated Capabilities:\nNone\n\nRemote-control command(s):\nMMEMory:DRIVes?"}, {"Level"=2, "Class Only"=FALSE, "Identifier"="RSSCOPE_ATTR_CHANGE_DRIVE", "Descriptive Name"="Change Drive", "Data Type"=2, "Command"="MMEM:MSIS", "Access"=1, "Range Table"="", "Read Callback"="", "Write Callback"="", "Supported Models"="", "Instrument Options"="", "Flags"=0, "Help"="Change current drive.\n\nAvailable Repeated Capabilities:\nNone\n\nRemote-control command(s):\nMMEMory:MSIS"}, {"Level"=2, "Class Only"=FALSE, "Identifier"="RSSCOPE_ATTR_CURRENT_DIRECTORY", "Descriptive Name"="Current Directory", "Data Type"=2, "Command"="MMEM:CDIR", "Access"=2, "Range Table"="", "Read Callback"="", "Write Callback"="", "Supported Models"="", "Instrument Options"="", "Flags"=0, "Help"="Changes the default directory for mass memory storage.\n\nAvailable Repeated Capabilities:\nNone\n\nRemote-control command(s):\nMMEMory:CDIRectory"}, {"Level"=2, "Class Only"=FALSE, "Identifier"="RSSCOPE_ATTR_CREATE_DIRECTORY", "Descriptive Name"="Create Directory", "Data Type"=2, "Command"="MMEM:MDIR", "Access"=1, "Range Table"="", "Read Callback"="", "Write Callback"="", "Supported Models"="", "Instrument Options"="", "Flags"=0, "Help"="Creates a new directory for mass memory storage.\n\nAvailable Repeated Capabilities:\nNone\n\nRemote-control command(s):\nMMEMory:MDIRectory"}, {"Level"=2, "Class Only"=FALSE, "Identifier"="RSSCOPE_ATTR_REMOVE_DIRECTORY", "Descriptive Name"="Remove Directory", "Data Type"=2, "Command"="MMEM:RDIR", "Access"=1, "Range Table"="", "Read Callback"="", "Write Callback"="", "Supported Models"="", "Instrument Options"="", "Flags"=0, "Help"="Removes an existing directory from the mass memory storage system.\n\nAvailable Repeated Capabilities:\nNone\n\nRemote-control command(s):\nMMEMory:RDIRectory"}, {"Level"=2, "Class Only"=FALSE, "Identifier"="RSSCOPE_ATTR_DELETE_FILE", "Descriptive Name"="Delete File", "Data Type"=2, "Command"="MMEM:DEL", "Access"=1, "Range Table"="", "Read Callback"="", "Write Callback"="", "Supported Models"="", "Instrument Options"="", "Flags"=0, "Help"="Removes a file from the specified directory.\n\nAvailable Repeated Capabilities:\nNone\n\nRemote-control command(s):\nMMEMory:DELete"}, {"Level"=2, "Class Only"=FALSE, "Identifier"="RSSCOPE_ATTR_SAVESET_PREVIEW_IMAGE", "Descriptive Name"="Saveset Preview Image", "Data Type"=3, "Command"="SAV:CONF:PREV", "Access"=2, "Range Table"="", "Read Callback"="", "Write Callback"="", "Supported Models"="", "Instrument Options"="", "Flags"=0, "Help"="If set to Off, the saveset is stored without the preview image to reduce the file size. Use this function each time before you save a saveset.\n\nAvailable Repeated Capabilities:\nNone\n\nRemote-control command(s):\nSAVeset:CONFig:PREView"}, {"Level"=2, "Class Only"=FALSE, "Identifier"="RSSCOPE_ATTR_SAVESET_ONE_FILE_NAME", "Descriptive Name"="Saveset One File Name", "Data Type"=2, "Command"="SAV:ONEF:NAME", "Access"=2, "Range Table"="", "Read Callback"="", "Write Callback"="", "Supported Models"="", "Instrument Options"="", "Flags"=0, "Help"="Sets the path and the file name of the One File. The file format is ZIP.\n\nAvailable Repeated Capabilities:\nNone\n\nRemote-control command(s):\nSAVeset:ONEFile:NAME"}, {"Level"=2, "Class Only"=FALSE, "Identifier"="RSSCOPE_ATTR_SAVESET_ONE_FILE_OPEN", "Descriptive Name"="Saveset One File Open", "Data Type"=4, "Command"="SAV:ONEF:OPEN", "Access"=1, "Range Table"="", "Read Callback"="", "Write Callback"="", "Supported Models"="", "Instrument Options"="", "Flags"=0, "Help"="Loads the One File that is specified with RSSCOPE_ATTR_SAVESET_ONE_FILE_NAME.\n\nAvailable Repeated Capabilities:\nNone\n\nRemote-control command(s):\nSAVeset:ONEFile:OPEN"}, {"Level"=2, "Class Only"=FALSE, "Identifier"="RSSCOPE_ATTR_SAVESET_ONE_FILE_SAVE", "Descriptive Name"="Saveset One File Save", "Data Type"=4, "Command"="SAV:ONEF:SAVE", "Access"=1, "Range Table"="", "Read Callback"="", "Write Callback"="", "Supported Models"="", "Instrument Options"="", "Flags"=0, "Help"="Saves the One File data to the file that is specified with RSSCOPE_ATTR_SAVESET_ONE_FILE_NAME.\n\nAvailable Repeated Capabilities:\nNone\n\nRemote-control command(s):\nSAVeset:ONEFile:SAVE"}, {"Level"=2, "Class Only"=TRUE, "Identifier"="", "Descriptive Name"="Waveform Export", "Data Type"=0, "Command"="", "Access"=0, "Range Table"="", "Read Callback"="", "Write Callback"="", "Supported Models"="", "Instrument Options"="", "Flags"=0, "Help"="This class attributes configures the storage settings for waveform data."}, {"Level"=3, "Class Only"=FALSE, "Identifier"="RSSCOPE_ATTR_WAVEFORM_EXPORT_MULTICHANNEL", "Descriptive Name"="Waveform Export Multichannel", "Data Type"=3, "Command"="EXP:WAV:MULT", "Access"=2, "Range Table"="", "Read Callback"="", "Write Callback"="", "Supported Models"="", "Instrument Options"="", "Flags"=0, "Help"="Enables or disables the multichannel export.\n\nAvailable Repeated Capabilities:\nNone\n\nRemote-control command(s):\nEXPort:WAVeform:MULTichannel"}, {"Level"=3, "Class Only"=FALSE, "Identifier"="RSSCOPE_ATTR_WAVEFORM_EXPORT_SOURCE", "Descriptive Name"="Waveform Export Source", "Data Type"=0, "Command"="EXP:WAV:SOUR", "Access"=2, "Range Table"="rsscope_rngWaveformParameter", "Read Callback"="", "Write Callback"="", "Supported Models"="", "Instrument Options"="", "Flags"=0, "Help"="This attribute configures the source waveform for export from the active waveforms of input channels, math signals and reference waveforms.\n\nAvailable Repeated
